vi "Auto Move Straight.vi"(8 "Error In":errorcluster, 11 "Refnum's In":T1) -> (0 "Error Out":errorcluster, 3 "Refnum's Out":T1)   [LabVIEW 2017]
uses:
  <vilib>/Rock Robotics/WPI/ThirdParty/Phoenix-LabVIEW/Motor Controller/Get/CTRE_Phoenix_MotorController_GetSelectedSensorData.vi
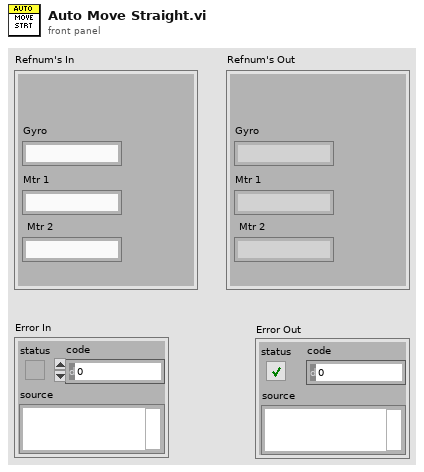
[diagram p1: front panel]
types:
  T1 = cluster{"Gyro":string, "Mtr 1":string, "Mtr 2":string}
  T2 = typedef "WPI_MotorControlDeviceRef.ctl" = cluster{"DeviceStatus":errorcluster, "Type":T3, "PWM":cluster{"PWM Channel":T4, "DeadBand":T5}, "CAN":cluster{"Device Number":u8, "SetOutput VI Ref":variant, "GetOutput VI Ref":variant, "Enable VI Ref":variant, "Disable VI Ref":variant, "Data":variant}, "Invert":bool, "DIO PWM":cluster{"PWM \"Enable\" Channel":T4, "DIOChannel":T6, "PWM Rate":dbl}}
  T3 = typedef "WPI_MotorControlType.ctl" = enum16{"PWM", "CAN", "DIO PWM"}
  T4 = typedef "FPGA_DIOPWMChannel.ctl" = enum8{"PWM 0", "PWM 1", "PWM 2", "PWM 3", "PWM 4", "PWM 5", "PWM 6", "PWM 7", "PWM 8", "PWM 9", "PWM MXP 0", "PWM MXP 1", "PWM MXP 2", "PWM MXP 3", "PWM MXP 4", "PWM MXP 5", "PWM MXP 6", "PWM MXP 7", "PWM MXP 8", "PWM MXP 9", "Invalid"}
  T5 = typedef "WPI_PWMDeadband.ctl" = cluster{"Name":string, "maxPositivePwm":i32, "minPositivePwm":i32, "centerPwm":i32, "maxNegativePwm":i32, "minNegativePwm":i32, "angularRange":u16}
  T6 = typedef "FPGA_DIOChannel.ctl" = enum8{"DIO 0", "DIO 1", "DIO 2", "DIO 3", "DIO 4", "DIO 5", "DIO 6", "DIO 7", "DIO 8", "DIO 9", "DIO MXP 0", "DIO MXP 1", "DIO MXP 2", "DIO MXP 3", "DIO MXP 4", "DIO MXP 5", "DIO MXP 6", "DIO MXP 7", "DIO MXP 8", "DIO MXP 9", "DIO MXP 10", "DIO MXP 11", "DIO MXP 12", "DIO MXP 13", "DIO MXP 14", "DIO MXP 15", "SPI Port CS1", "SPI Port CS2", "SPI Port CS3", "SPI Port MISO", "SPI Port MOSI", "Invalid"}
  T7 = typedef "WPI_GyroDevRef.ctl" = cluster{"DevStatus":errorcluster, "Analog Channel":T8, "Gain (VoltsPerDegree/Second)":dbl, "Gyro Type":enum16{"Analog", "XRS450"}, "Handle":i32, "SPI Bus":T9, "Device Found":bool, "Sample Rate":dbl, "Calibrate On Open":bool, "Offset":dbl}
  T8 = typedef "FPGA_AIChannel.ctl" = enum8{"AI 0", "AI 1", "AI 2", "AI 3", "AI MXP 0", "AI MXP 1", "AI MXP 2", "AI MXP 3", "Invalid"}
  T9 = typedef "spi_bus.ctl" = enum16{"SPI On-Board, CS0", "SPI On-Board, CS1", "SPI On-Board, CS2", "SPI On-Board, CS3", "SPI MXP", "Invalid"}
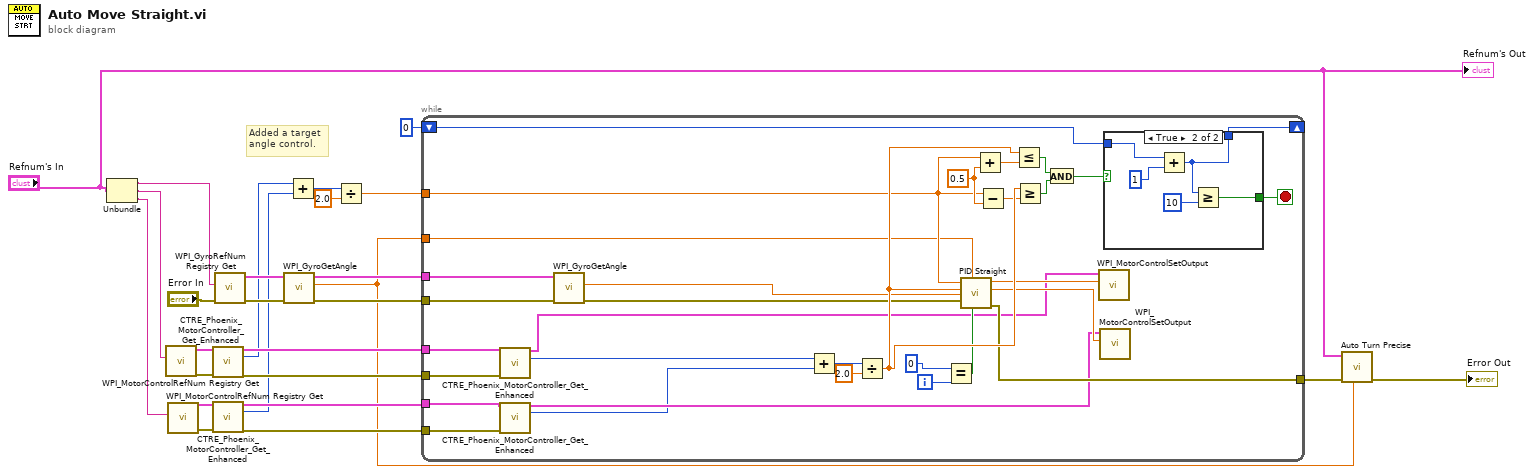
[diagram p0: block diagram]
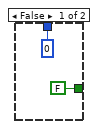
[diagram p2: hidden frame]
diagram:
  # "Added a target\nangle control."
  n1 = Unbundle("Refnum's In") -> ("Gyro"=w17:string, "Mtr 1"=w16:string, "Mtr 2"=w15:string)
  n2 = call <vilib>:"WPI_MotorControlRefNum Registry Get.vi"("refnum name"=w16) -> ("error out"=w11:errorcluster, "MotorControlDevRef"=w14:T2)  [unwired: 9 in]
  n3 = call <vilib>:"WPI_MotorControlRefNum Registry Get.vi"("refnum name"=w15) -> ("error out"=w9:errorcluster, "MotorControlDevRef"=w10:T2)  [unwired: 9 in]
  n4 = call-poly <vilib>:"CTRE_Phoenix_MotorController_Get_Enhanced.vi"("PhoenixMotorControlDevRef"=w14, "error in"=w11) -> ("PhoenixMotorControlDevRef"=w13:T2, "Position (Raw Sensor Units)"=w4:i32, "error out"=w12:errorcluster)  [unwired: 10 in, 1 out]
  n5 = call-poly <vilib>:"CTRE_Phoenix_MotorController_Get_Enhanced.vi"("PhoenixMotorControlDevRef"=w10, "error in"=w9) -> ("PhoenixMotorControlDevRef"=w8:T2, "Position (Raw Sensor Units)"=w3:i32, "error out"=w7:errorcluster)  [unwired: 10 in, 1 out]
  n6 = call <vilib>:"WPI_GyroRefNum Registry Get.vi"("error in (no error)"="Error In", "refnum name"=w17) -> ("error out"=w20:errorcluster, "GyroDevRef"=w19:T7)  [unwired: 8 in]
  n7 = call <vilib>:"WPI_GyroGetAngle.vi"("error in"=w20, "GyroDevRef"=w19) -> ("error out"=w22:errorcluster, "Angle"=w1:dbl, "GyroDevRef"=w21:T7)  [unwired: 5 in, 2 out]
  n8 = Add(x=w4, y=w3) -> (x+y=w5:i32)
  n9 = Divide(x=w5, y=2.0) -> (x/y=w2:dbl)
  n10 = while {
    shift-right: [w47] -> _
    shift-left: 0 -> [w46]
    tunnel: w2 -> [w36]
    tunnel: [w42] -> w25
    tunnel: w1 -> [w35]
    tunnel: w21 -> [w38]
    tunnel: w22 -> [w37]
    tunnel: w8 -> [w34]
    tunnel: w7 -> [w33]
    tunnel: w13 -> [w28]
    tunnel: w12 -> [w27]
    i -> [w58]
    stop <- w41 stop-if-true
    w54 = 0.5 ("y")
    n11 = call-poly <vilib>:"CTRE_Phoenix_MotorController_Get_Enhanced.vi"("PhoenixMotorControlDevRef"=w28, "error in"=w27) -> ("PhoenixMotorControlDevRef"=w29:T2, "Position (Raw Sensor Units)"=w30:i32)  [unwired: 10 in, 2 out]
    n12 = call-poly <vilib>:"CTRE_Phoenix_MotorController_Get_Enhanced.vi"("PhoenixMotorControlDevRef"=w34, "error in"=w33) -> ("PhoenixMotorControlDevRef"=w32:T2, "Position (Raw Sensor Units)"=w31:i32)  [unwired: 10 in, 2 out]
    n13 = call <vilib>:"WPI_GyroGetAngle.vi"("error in"=w37, "GyroDevRef"=w38) -> ("error out"=w43:errorcluster, "Angle"=w45:dbl)  [unwired: 5 in, 3 out]
    n14 = Add(x=w30, y=w31) -> (x+y=w55:i32)
    n15 = Divide(x=w55, y=2.0) -> (x/y=w52:dbl)
    n16 = Equal?(x=0, y=w58) -> (x = y?=w44:bool)
    n17 = call "PID Straight.vi"("Reinitialize"=w44, "Target Angle"=w35, "Error In"=w43, "Gyro Angle"=w45, "Current Distance"=w52, "Target Distance"=w36) -> ("Error Out"=w42:errorcluster, "Right Power"=w39:dbl, "Left Power"=w40:dbl)  [unwired: 3 in]
    n18 = Add(x=w36, y=w54) -> (x+y=w53:dbl)
    n19 = Subtract(x=w36, y=w54) -> (x-y=w51:dbl)
    n20 = Less Or Equal?(x=w52, y=w53) -> (x <= y?=w50:bool)
    n21 = Greater Or Equal?(x=w52, y=w51) -> (x >= y?=w49:bool)
    n22 = And(x=w50, y=w49) -> (x .and. y?=w48:bool)
    n23 = call <vilib>:"WPI_MotorControlSetOutput.vi"("Output"=w40, "MotorControlDevRef"=w29) -> ()  [unwired: 7 in, 3 out]
    n24 = call <vilib>:"WPI_MotorControlSetOutput.vi"("Output"=w39, "MotorControlDevRef"=w32) -> ()  [unwired: 7 in, 3 out]
    n25 = case shown="True" w48 {
      tunnel: w46 -> [_ w64]
      tunnel: [0 w63] -> w47
      tunnel: [FALSE w61] -> w41
      frame False {
      }
      frame True {
        n26 = Add(x=w64, y=1) -> (x+y=w63:i32)
        n27 = Greater Or Equal?(x=w63, y=10) -> (x >= y?=w61:bool)
      }
    }
  }
  n28 = call "Auto Turn Precise.vi"("Target Distance"=w1, "Error In"=w25, "Refnum's In"="Refnum's In") -> ("Error Out"=→"Error Out":errorcluster)  [unwired: 7 in, 1 out]
  "Refnum's Out" <- "Refnum's In"
